vi "zapiszWspolrzednePoziome.vi"(9 "Nowy nr pozycji poziomej":i32, 10 "Wybor komory":T1, 11 "Lista punkow w poziomie":i32[](array[numeric])) -> ()   [LabVIEW 2014]
uses:
  parametryKomorVIs/WyborKomory.ctl
  AkcjaGFV.ctl
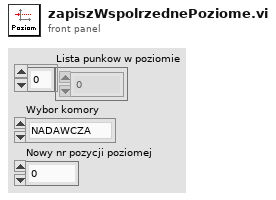
[diagram p1: front panel]
types:
  T1 = typedef "WyborKomory.ctl" = enum16{"NADAWCZA", "ODBIORCZA"}
  T2 = typedef "AkcjaGFV.ctl" = enum16{"Czytaj", "Zapisz", "Reset"}
  T3 = typedef "WyjsciaParametry.ctl" = cluster{"Nad. lewo":bool, "Nad.  prawo":bool, "Nad.  gora":bool, "Nad. do³":bool, "Dzialanie":bool, "Pomiar":bool, "Odb. lewo":bool, "Odb.  prawo":bool, "Odb.  gora":bool, "Odb. dol":bool, "Pozostalo punktow":i32, "Nad. elewacja":i32, "Nad. azymut":i32, "Odb. elewacja":i32, "Odb. azymut":i32, "TCP Error":bool, "TCP Error Code":i32, "LINX Error":bool, "LINX Error Code":i32, "Nastepny elewacja":i32, "Nastepny azymut":i32, "Coords Error":bool, "Inicjalizacja pozycji":bool, "Generator Error":bool, "Error Code":i32}
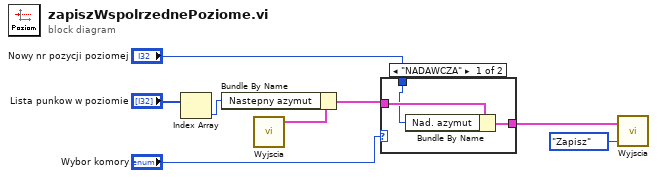
[diagram p0: block diagram]
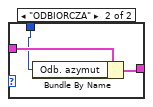
[diagram p2: hidden frame]
diagram:
  n1 = Index Array(array="Lista punkow w poziomie") -> (element=w8:i32)  [unwired: 1 in]
  n2 = call "Wyjscia.vi"() -> ("Wyjœcie"=w7:T3)  [unwired: 5 in]
  n3 = Bundle By Name(cluster=w7, "Nastepny azymut"=w8) -> (w4:T3)
  n4 = case shown="\"NADAWCZA\"" "Wybor komory" {
    tunnel: "Nowy nr pozycji poziomej" -> [w10 w12]
    tunnel: w4 -> [w11 w13]
    tunnel: [w9 w14] -> w1
    frame "NADAWCZA" {
      n5 = Bundle By Name(cluster=w11, "Nad. azymut"=w10) -> (w9:T3)
    }
    frame "ODBIORCZA" {
      n6 = Bundle By Name(cluster=w13, "Odb. azymut"=w12) -> (w14:T3)
    }
  }
  n7 = call "Wyjscia.vi"("Akcja"=AkcjaGFV."Zapisz", "Wejœcie"=w1) -> ()  [unwired: 3 in, 1 out]
